vi "array sales ex 4.vi"() -> ()   [LabVIEW 2020]
panel:
  out "size(s)":i32[](array[numeric])
  out "COLUMN SUM":dbl
  out "subarray 2":string[](array[string])
  out "SEARCH SALES DATA ARRAY":string[][](array[string])
  in  "Search Value":string
  out "subarray":string[](array[string])
  in  "COLUMN HEADING":T1(ring)
  out "sales data":string[][](array[string])
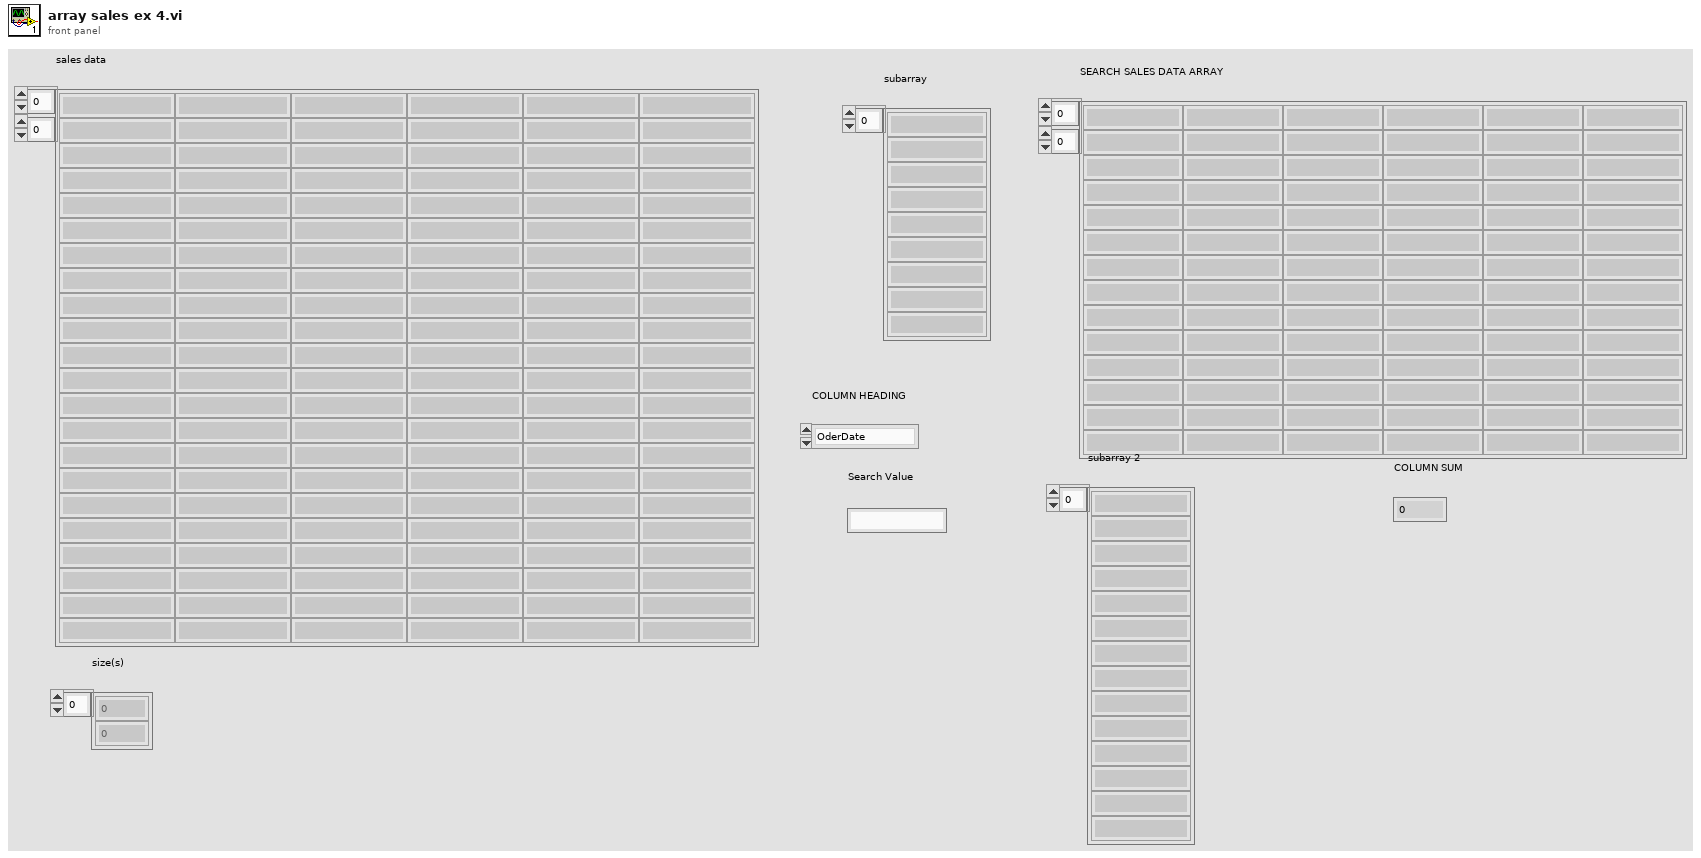
[diagram p1: front panel]
types:
  T1 = enum16{"OderDate", "Region", "Rep", "Item", "Units", "UnitCost"}
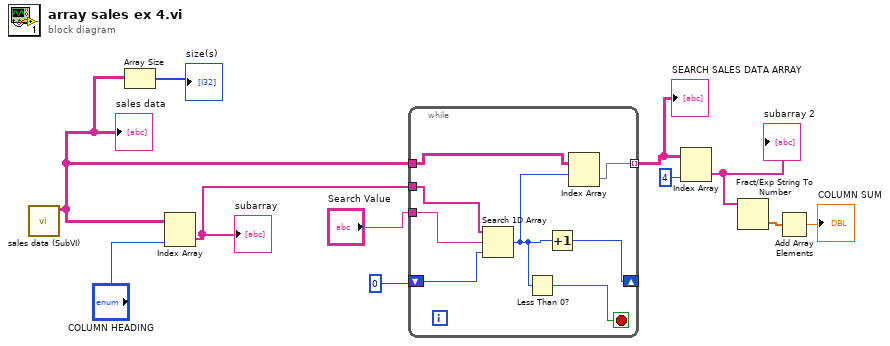
[diagram p0: block diagram]
diagram:
  n1 = call "sales data (SubVI).vi"() -> ("sales data"=w3:string[][])  [unwired: 11 in]
  "sales data" <- w3
  n2 = Array Size(array=w3) -> (size(s)=→"size(s)":i32[])
  n3 = Index Array(array=w3, index (col)="COLUMN HEADING") -> (element=w11:string[])  [unwired: 1 in]
  "subarray" <- w11
  n4 = while {
    tunnel: w11 -> [w17]
    tunnel: "Search Value" -> [w16]
    tunnel: w3 -> [w19]
    tunnel: [w18] -> w9 mode=indexing
    shift-right: [w14] -> _
    shift-left: 0 -> [w15]
    stop <- w12 stop-if-true
    n5 = Search 1D Array(1D array=w17, element=w16, start index (0)=w15) -> (index of element=w13:i32)
    n6 = Less Than 0?(x=w13) -> (x < 0?=w12:bool)
    n7 = Increment(x=w13) -> (x+1=w14:i32)
    n8 = Index Array(array=w19, index (row)=w13) -> (element=w18:string[])  [unwired: 1 in]
  }
  "SEARCH SALES DATA ARRAY" <- w9
  n9 = Index Array(array=w9, index (col)=4 ("disabled index (col)")) -> (element=w6:string[])  [unwired: 1 in]
  "subarray 2" <- w6
  n10 = Fract/Exp String To Number(string=w6) -> (number=w5:dbl[])  [unwired: 3 in, 1 out]
  n11 = Add Array Elements(numeric array=w5) -> (sum=→"COLUMN SUM":dbl)
